vi "RT Driver VI.vi"(7 "Operation":T1, 11 "Device Reference in":T2 format="%.0x") -> (0 "Error Code":i32)   [LabVIEW 2015, in "SLSC Module Template Engine.lvlib"]
uses:
  SLSC Module Template Engine.lvlib
  <vilib>/NI Veristand/Custom Device API/Custom Device Item Ref.ctl
  <vilib>/NI Veristand/Custom Device API/Hardware Interface Driver VI Operation.ctl
  Shared/Compiled.Settings
  Shared/SLSC Dynamic Channel.ctl
  Types/RTStateVariables.ctl
  <vilib>/NI/NIVS Inline Async API/_VS Inline Async API/VS Inline Async API/VS Inline Async API.lvclass
  <vilib>/NI/NIVS Inline Async API/_VS Inline Async API/VS Inline Async API/VS Inline Async API.lvclass/VS Inline Async API.ctl
  <vilib>/NI/NIVS Inline Async API/_Data Access Engine/Data Access Engine/Data Access Engine.lvclass/Data Access Engine.ctl
  <vilib>/NI/NIVS Inline Async API/_Data Access Engine/Access Type Classes/Write/Write.lvclass/Write.ctl
  <vilib>/NI/NIVS Inline Async API/_Data Access Engine/Access Type Classes/ReadWrite/ReadWrite.lvclass/ReadWrite.ctl
  <vilib>/NI/NIVS Inline Async API/_Data Access Engine/Access Type Classes/Read/Read.lvclass/Read.ctl
  <vilib>/NI/NIVS Inline Async API/_Data Access Engine/Data Access Engine/Methods/Data.Engine.Read Data from HW.vi
  <vilib>/NI/NIVS Inline Async API/_VS Inline Async API/Error Handling Process/SubVIs/Error.GetError.vi
  <vilib>/NI/NIVS Inline Async API/_Data Access Engine/Data Access Engine/Methods/Data.Engine.Write Data to HW.vi
  <vilib>/NI/NIVS Inline Async API/_Data Access Engine/Access Type Classes/ReadWrite/ReadWrite.EngineData.vi
  <vilib>/NI/NIVS Inline Async API/_Data Access Engine/Access Type Classes/Write/Write.EngineData.vi
  <vilib>/NI/NIVS Inline Async API/_Data Access Engine/Access Type Classes/Read/Read.EngineData.vi
  <vilib>/NI Veristand/Custom Device API/NI VeriStand - Get Channel Value by Data Reference.vi
  <vilib>/NI Veristand/Custom Device API/NI VeriStand - Set Channel Value by Data Reference.vi
  <vilib>/NI Veristand/Custom Device API/NI VeriStand - Get Channel Values by Block Data Reference.vi
  Shared/Constants.vi
  <vilib>/NI Veristand/Custom Device API/Get Item Property (Variant).vi
  <vilib>/SLSC/Initialize Session without Resources.vi
  <vilib>/SLSC/Close Session.vi
  <vilib>/NI Veristand/Custom Device API/Global Data Refs.vi
  <vilib>/NI VeriStand/Custom Device API/Custom Device API.lvlib
  Shared/SLSC Module Template Shared.lvlib
  <vilib>/NI Veristand/Custom Device Tools/Custom Device Utility Library/Custom Device Utility Library.lvlib
  System Explorer/SLSC Module Template System Explorer.lvlib
  <vilib>/SLSC/SLSC.lvlib
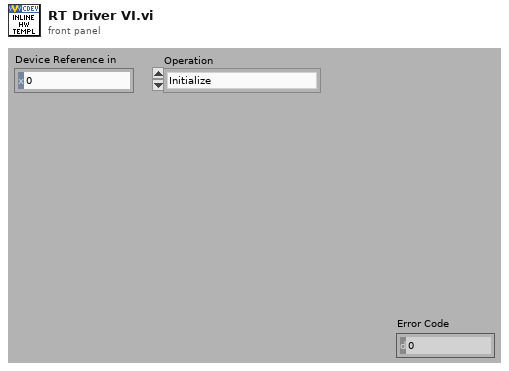
[diagram p1: front panel]
types:
  T1 = typedef "Custom Device API.lvlib/Hardware Interface Driver VI Operation.ctl" = enum16{"Initialize", "Start", "Read Data from HW", "Write Data to HW", "Close"}
  T2 = typedef "Custom Device API.lvlib/Custom Device Item Ref.ctl" = u64
  T3 = typedef "SLSC Module Template Engine.lvlib/RTStateVariables.ctl" = cluster{"Async":refnum<class "VS Inline Async API.lvclass">, "Settings":T4}
  T4 = typedef "SLSC Module Template Shared.lvlib/Compiled.Settings" = cluster{"Name":string, "SLSC IP Address":string, "Slot #":i32, "Configuration Data":cluster{"Properties":cluster{"Boolean Properties":cluster{"property":refnum<k21>, "Value":bool, "SLSC Item":refnum<k21>}[], "Double Properties":cluster{"property":refnum<k21>, "Double Write":dbl, "SLSC Item":refnum<k21>}[], "I32 Properties":cluster{"property":refnum<k21>, "Int32 Write":i32, "SLSC Item":refnum<k21>}[], "I64 Properties":cluster{"property":refnum<k21>, "Int64 Write":i64, "SLSC Item":refnum<k21>}[], "String Properties":cluster{"property":refnum<k21>, "String Write":string, "SLSC Item":refnum<k21>}[], "U32 Properties":cluster{"property":refnum<k21>, "UInt32 Write":u32, "SLSC Item":refnum<k21>}[], "U64 Properties":cluster{"property":refnum<k21>, "UInt64 Write":u64, "SLSC Item":refnum<k21>}[]}}, "SLSC Dynamic Inputs":T5[], "SLSC Dynamic Outputs":T5[], "SLSC Dynamic Commands":T5[]}
  T5 = typedef "SLSC Module Template System Explorer.lvlib/SLSC Dynamic Channel.ctl" = cluster{"SLSC Item":string, "property":string, "Data Type":enum16{"Bool", "Double", "I32", "I64", "String", "U32", "U64"}}
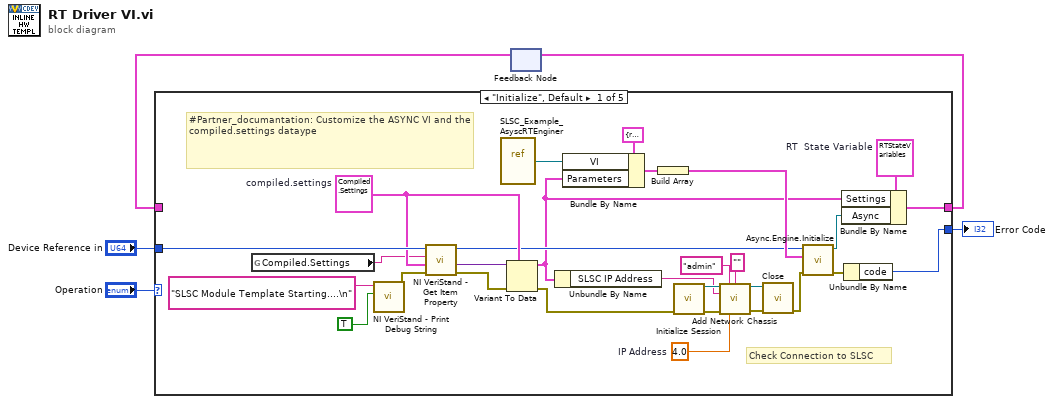
[diagram p0: block diagram]
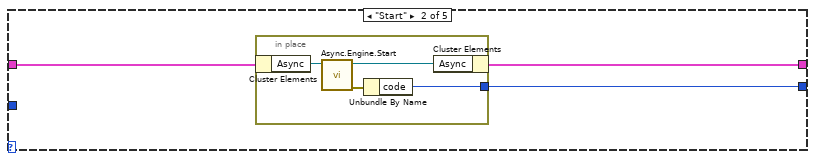
[diagram p2: hidden frame]
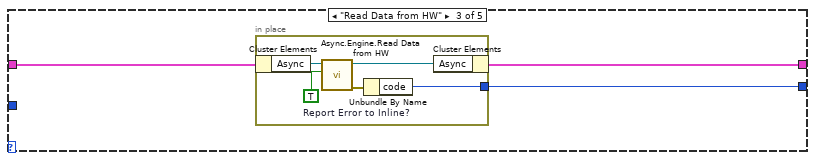
[diagram p3: hidden frame]
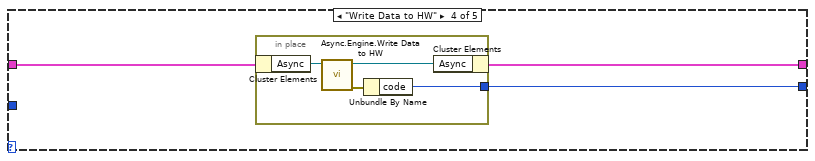
[diagram p4: hidden frame]
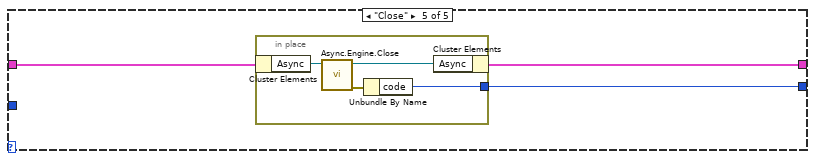
[diagram p5: hidden frame]
diagram:
  n1 = feedback #1() -> (w3:T3)  [unwired: 1 out]
  n2 = case shown="\"Initialize\", Default" "Operation" {
    tunnel: [w32 w36 w42 w50 w58] -> w4
    tunnel: w3 -> [_ w37 w44 w51 w59]
    tunnel: "Device Reference in" -> [w29 _ _ _ _]
    tunnel: [w34 w35 w43 w52 w57] -> w1
    frame "Initialize", Default {
      w13 = 4.0  # IP Address
      w24 = T3 {"Async"=refnum, "Settings"={"Name"="", "SLSC IP Address"="", "Slot #"=0, "Configuration Data"={"Properties"={"Boolean Properties"=[], "Double Properties"=[], "I32 Properties"=[], "I64 Properties"=[], "String Properties"=[], "U32 Properties"=[], "U64 Properties"=[]}}, "SLSC Dynamic Inputs"=[], "SLSC Dynamic Outputs"=[], "SLSC Dynamic Commands"=[]}}  # RT  State Variable
      w25 = T4 {"Name"="", "SLSC IP Address"="", "Slot #"=0, "Configuration Data"={"Properties"={"Boolean Properties"=[], "Double Properties"=[], "I32 Properties"=[], "I64 Properties"=[], "String Properties"=[], "U32 Properties"=[], "U64 Properties"=[]}}, "SLSC Dynamic Inputs"=[], "SLSC Dynamic Outputs"=[], "SLSC Dynamic Commands"=[]}  # compiled.settings
      # "Check Connection to SLSC"
      # "#Partner_documantation: Customize the ASYNC VI and the compiled.settings dataype"
      n3 = global read "Constants.vi" "Compiled.Settings"() -> (w19:string)
      n4 = call <vilib>:"NI VeriStand - Print Debug String.vi"("Add to log file? (T)"=TRUE, "Message"="SLSC Module Template Starting....\n") -> ("error out"=w21:errorcluster)  [unwired: 9 in]
      n5 = call-poly <vilib>:"NI VeriStand - Get Item Property.vi"("error in (no error)"=w21, "Default Value"=w25, "Property Name"=w19, "Item Ref in"=w29) -> ("error out"=w28:errorcluster, "Value"=w27:variant, "Item Ref out"=w22:T2)  [unwired: 4 in, 1 out]
      n6 = vi-ref "SLSC_Example_AsyscRTEnginer.vi"() -> (w17:refnum<vi>)
      n7 = Variant To Data(error in=w28, type=w25, Variant=w27) -> (data=w16:T4, error out=w6:errorcluster)
      n8 = Unbundle By Name(w16) -> ("SLSC IP Address"=w7:string)
      n9 = Bundle By Name(cluster=cluster{"VI":refnum<vi>, "Parameters":variant} {"VI"=refnum, "Parameters"=variant} ("Process"), "VI"=w17, "Parameters"=w16) -> (w30:cluster{"VI":refnum<vi>, "Parameters":variant})
      n10 = Build Array(w30) -> (w23:cluster{"VI":refnum<vi>, "Parameters":variant}[])
      n11 = call-poly <vilib>:"Initialize Session.vi"("error in (no error)"=w6) -> ("session out"=w12:refnum<k21>, "error out"=w14:errorcluster)  [unwired: 13 in]
      n12 = call <vilib>:"Add Network Chassis.vi"("session in"=w12, "username"="admin" ("Username"), "password"="" ("Password"), "chassis IP address/hostname"=w7, "error in (no error)"=w14, "connect timeout (60 sec)"=w13) -> ("session out"=w11:refnum<k21>, "error out"=w10:errorcluster)  [unwired: 7 in, 1 out]
      n13 = call-poly <vilib>:"Close.vi"("session in"=w11, "error in (no error)"=w10) -> ("error out"=w15:errorcluster)  [unwired: 13 in]
      n14 = call <vilib>:"Async.Engine.Initialize.vi"("error in (no error)"=w15, "Processes"=w23, "Custom Device Ref"=w22) -> ("error out"=w26:errorcluster, "Async"=w33:refnum<class "VS Inline Async API.lvclass">)  [unwired: 7 in]
      n15 = Bundle By Name(cluster=w24, "Settings"=w16, "Async"=w33) -> (w32:T3)
      n16 = Unbundle By Name(w26) -> ("code"=w34:i32)
    }
    frame "Start" {
      n17 = in-place {
        in-place-border: [w38] -> w35
        n18 = in-place-cluster #2(w37) -> ("Async"=w41:refnum<class "VS Inline Async API.lvclass">)
        n19 = call <vilib>:"Async.Engine.Start.vi"("VS Inline Async API in"=w41) -> ("error out"=w39:errorcluster, "VS Inline Async API out"=w40:refnum<class "VS Inline Async API.lvclass">)  [unwired: 9 in]
        n20 = Unbundle By Name(w39) -> ("code"=w38:i32)
        n21 = in-place-cluster #2("Async"=w40) -> (w36:T3)
      }
    }
    frame "Read Data from HW" {
      n22 = in-place {
        in-place-border: [w47] -> w43
        w45 = TRUE  # Report Error to Inline?
        n23 = in-place-cluster #3(w44) -> ("Async"=w49:refnum<class "VS Inline Async API.lvclass">)
        n24 = call <vilib>:"Async.Engine.Read Data from HW.vi"("Report Error to Inline?"=w45, "Async in"=w49) -> ("error out"=w46:errorcluster, "Async out"=w48:refnum<class "VS Inline Async API.lvclass">)  [unwired: 8 in]
        n25 = Unbundle By Name(w46) -> ("code"=w47:i32)
        n26 = in-place-cluster #3("Async"=w48) -> (w42:T3)
      }
    }
    frame "Write Data to HW" {
      n27 = in-place {
        in-place-border: [w56] -> w52
        n28 = in-place-cluster #4(w51) -> ("Async"=w54:refnum<class "VS Inline Async API.lvclass">)
        n29 = call <vilib>:"Async.Engine.Write Data to HW.vi"("VS Inline Async API in"=w54) -> ("error out"=w55:errorcluster, "VS Inline Async API out"=w53:refnum<class "VS Inline Async API.lvclass">)  [unwired: 9 in]
        n30 = Unbundle By Name(w55) -> ("code"=w56:i32)
        n31 = in-place-cluster #4("Async"=w53) -> (w50:T3)
      }
    }
    frame "Close" {
      n32 = in-place {
        in-place-border: [w61] -> w57
        n33 = in-place-cluster #5(w59) -> ("Async"=w63:refnum<class "VS Inline Async API.lvclass">)
        n34 = call <vilib>:"Async.Engine.Close.vi"("Async in"=w63) -> ("error out"=w60:errorcluster, "Async out"=w62:refnum<class "VS Inline Async API.lvclass">)  [unwired: 9 in]
        n35 = Unbundle By Name(w60) -> ("code"=w61:i32)
        n36 = in-place-cluster #5("Async"=w62) -> (w58:T3)
      }
    }
  }
  "Error Code" <- w1
  n37 = feedback-in #1(w4) -> ()
